vi "PFD_AirspeedSpeed.vi"(8 "Refresh Rate (Hz)":u32=30) -> ()   [LabVIEW 2023]
uses:
  pfd_global.vi
panel:
  out "AIRSPEED":bool
  out "PFD_AirSpeedControl":sgl
  out "PFD_Airspeed":picture
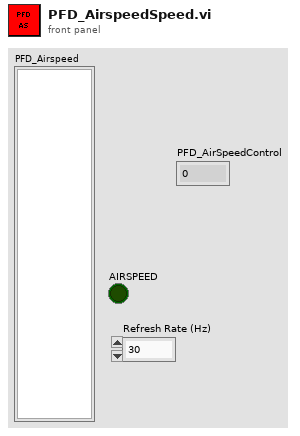
[diagram p1: front panel]
types:
  T1 = cluster{"left":i16, "top":i16, "right":i16, "bottom":i16}
  T2 = cluster{"horizontal":enum16{"left", "center", "right"}, "vertical":enum16{"top", "center", "bottom"}}
  T3 = enum16{"User-specified Font", "Application Font", "System Font", "Dialog Font"}
  T4 = cluster{"Font Name:":string, "Size":i16, "Strikeout?":bool, "Italic?":bool, "Underline?":bool, "Outline?":bool, "Shadow?":bool, "Bold?":bool}
  T5 = cluster{cluster{"Width 3":i16, i16}, cluster{"Width 4":i16, i16}}
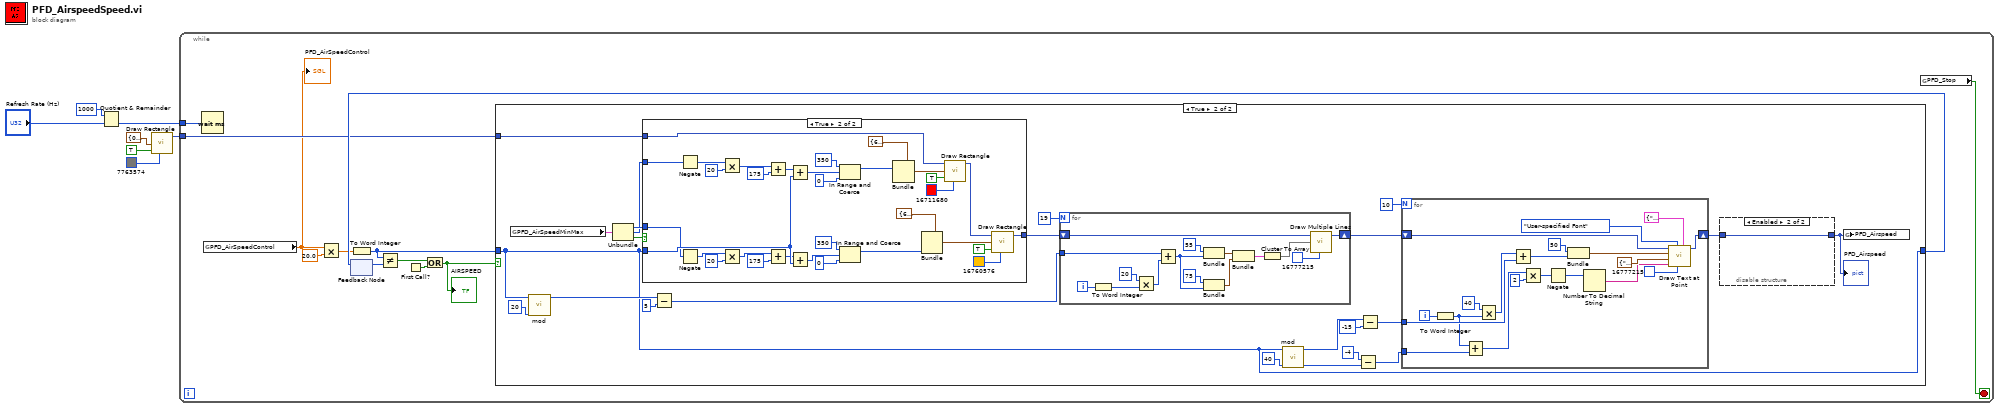
[diagram p0: block diagram]
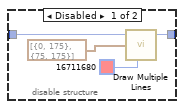
[diagram p3: hidden frame]
diagram:
  n1 = Quotient & Remainder(x=u32 1000, y="Refresh Rate (Hz)") -> (floor(x/y)=w1:u32)  [unwired: 1 out]
  n2 = call <vilib>:"Draw Rectangle.vi"("rect"=T1 {"left"=0, "top"=0, "right"=75, "bottom"=350}, "fill?(F)"=TRUE, "color(black)"=u32 7763574 ("Speed_color_background")) -> ("new picture"=w7:picture)  [unwired: 6 in]
  n3 = while {
    tunnel: w7 -> [w15]
    tunnel: w1 -> [w11]
    stop <- w9 stop-if-true
    n4 = Wait (ms)(milliseconds to wait=w11) -> ()  [unwired: 1 out]
    n5 = global read "pfd_global.vi" "PFD_AirSpeedControl"() -> (w10:sgl)
    "PFD_AirSpeedControl" <- w10
    n6 = Multiply(x=w10, y=sgl 20.0) -> (x*y=w12:sgl)
    n7 = To Word Integer(number=w12) -> (16bit integer=w13:i16)
    n8 = feedback #1() -> (w18:i16)  [unwired: 1 in]
    n9 = Not Equal?(x=w13, y=w18) -> (x != y?=w17:bool)
    n10 = First Call?() -> (First Call?: T/F=w16:bool)
    n11 = Or(x=w17, y=w16) -> (x .or. y?=w8:bool)
    "AIRSPEED" <- w8
    n12 = case shown="True" w8 {
      tunnel: [w20 w30] -> w19
      tunnel: w13 -> [w20 w30]
      tunnel: w15 -> [_ w39]
      frame False {
      }
      frame True {
        n13 = global read "pfd_global.vi" "PFD_AirSpeedMinMax"() -> (w35:cluster{"Max":i16, "Min":i16, "Show":bool})
        n14 = call "mod.vi"("Divide"=i16 20 ("x"), "Value In"=w30) -> ("Value out"=w43:i16)  [unwired: 8 in, 1 out]
        n15 = Unbundle(w35) -> ("Max"=w38:i16, "Min"=w37:i16, "Show"=w36:bool)
        n16 = case shown="True" w36 {
          tunnel: w30 -> [_ w99]
          tunnel: w37 -> [_ w71]
          tunnel: w38 -> [_ w91]
          tunnel: [w69 w100] -> w34
          tunnel: w39 -> [w69 w72]
          frame False {
          }
          frame True {
            n17 = Negate(x=w71) -> (-x=w70:i16)
            n18 = Negate(x=w91) -> (-x=w94:i16)
            n19 = Multiply(x=w70, y=i16 20) -> (x*y=w98:i16)
            n20 = Multiply(x=w94, y=i16 20) -> (x*y=w92:i16)
            n21 = Add(x=w98, y=i16 175 ("top")) -> (x+y=w97:i16)
            n22 = Add(x=w92, y=i16 175) -> (x+y=w93:i16)
            n23 = Add(x=w97, y=w99) -> (x+y=w78:i16)
            n24 = Add(x=w93, y=w99) -> (x+y=w74:i16)
            n25 = In Range and Coerce(upper limit=i16 350, x=w78, lower limit=i16 0) -> (coerced(x)=w77:i16)  [unwired: 1 out]
            n26 = In Range and Coerce(upper limit=i16 350, x=w74, lower limit=i16 0) -> (coerced(x)=w73:i16)  [unwired: 1 out]
            n27 = Bundle(cluster=T1 {"left"=60, "top"=175, "right"=76, "bottom"=350} ("rect"), "top"=w77) -> (w85:T1)  [unwired: 3 in]
            n28 = Bundle(cluster=T1 {"left"=60, "top"=0, "right"=76, "bottom"=75} ("rect 2"), "bottom"=w73) -> (w81:T1)  [unwired: 3 in]
            n29 = call <vilib>:"Draw Rectangle.vi"("picture"=w72, "rect"=w85, "fill?(F)"=TRUE, "color(black)"=u32 16711680) -> ("new picture"=w101:picture)  [unwired: 5 in]
            n30 = call <vilib>:"Draw Rectangle.vi"("picture"=w101, "rect"=w81, "fill?(F)"=TRUE, "color(black)"=u32 16760576) -> ("new picture"=w100:picture)  [unwired: 5 in]
          }
        }
        n31 = Subtract(x=w43, y=i16 5) -> (x-y=w40:i16)
        n32 = for {
          N: 19 ("Numeric") -> [_]
          shift-right: [w103] -> w32
          shift-left: w34 -> [w108]
          tunnel: w40 -> [w106]
          i -> [w107]
          n33 = To Word Integer(number=w107) -> (16bit integer=w102:i16)
          n34 = Multiply(x=i16 20, y=w102) -> (x*y=w110:i16)
          n35 = Add(x=w106, y=w110) -> (x+y=w104:i16)
          n36 = Bundle("Width 3"=i16 55, w104) -> (w115:cluster{"Width 3":i16, i16})  [unwired: 1 in]
          n37 = Bundle("Width 4"=i16 75, w104) -> (w114:cluster{"Width 4":i16, i16})  [unwired: 1 in]
          n38 = Bundle(w115, w114) -> (w116:T5)  [unwired: 1 in]
          n39 = Cluster To Array(cluster=w116) -> (array=w112:cluster{"Width 4":i16, i16}[])
          n40 = call <vilib>:"Draw Multiple Lines.vi"("picture"=w108, "line endpoints"=w112, "color(black)"=u32 16777215) -> ("new picture"=w103:picture)  [unwired: 6 in]
        }
        n41 = call "mod.vi"("Divide"=i16 40, "Value In"=w30) -> ("Ceil"=w24:i16, "Value out"=w27:i16)  [unwired: 8 in]
        n42 = Subtract(x=i16 -4, y=w24) -> (x-y=w25:i16)
        n43 = Subtract(x=w27, y=i16 -15) -> (x-y=w26:i16)
        n44 = for {
          N: 10 ("Numeric") -> [_]
          shift-right: [w65] -> w22
          shift-left: w32 -> [w66]
          tunnel: w26 -> [w55]
          tunnel: w25 -> [w54]
          i -> [w56]
          n45 = To Word Integer(number=w56) -> (16bit integer=w53:i16)
          n46 = Add(x=w53, y=w54) -> (x+y=w51:i16)
          n47 = Multiply(x=i16 40 ("Divide"), y=w53) -> (x*y=w60:i16)
          n48 = Add(x=w60, y=w55) -> (x+y=w59:i16)
          n49 = Multiply(x=w51, y=i16 2) -> (x*y=w50:i16)
          n50 = Negate(x=w50) -> (-x=w49:i16)
          n51 = Bundle("Width 3"=i16 50, w59) -> (w58:cluster{"Width 3":i16, i16})  [unwired: 1 in]
          n52 = Number To Decimal String(number=w49) -> (decimal integer string=w57:string)  [unwired: 1 in]
          n53 = call <vilib>:"Draw Text at Point.vi"("[user-specified font]"=T4 {"Font Name:"="a", "Size"=18, "Strikeout?"=FALSE, "Italic?"=FALSE, "Underline?"=FALSE, "Outline?"=FALSE, "Shadow?"=FALSE, "Bold?"=TRUE}, "text color(black)"=u32 16777215, "desired font(Application)"=T3."User-specified Font", "text"=w57, "alignment(left, top)"=T2 {"horizontal"=enum."right", "vertical"=enum."center"}, "origin"=w58, "picture"=w66) -> ("new picture"=w65:picture)  [unwired: 3 in, 1 out]
        }
        n54 = disable-structure shown="Enabled" {
          disable-tunnel: w22 -> [w47 w48]
          disable-tunnel: [w46 w48] -> w21
          frame Disabled {
            n55 = call <vilib>:"Draw Multiple Lines.vi"("picture"=w47, "line endpoints"=cluster{"x":i16, "y":i16}[] [{"x"=0, "y"=175}, {"x"=75, "y"=175}], "color(black)"=u32 16711680) -> ("new picture"=w46:picture)  [unwired: 6 in]
          }
          frame Enabled {
          }
        }
        "PFD_Airspeed" <- w21
        n56 = global write "pfd_global.vi" "PFD_Airspeed"(w21) -> ()
      }
    }
    n57 = feedback-in #1(w19) -> ()
    n58 = global read "pfd_global.vi" "PFD_Stop"() -> (w9:bool)
  }
